vi "Init GUI.vi"(8 "error in (no error)":errorcluster, 11 "Guardian in":refnum<class "Guardian.lvclass">) -> (0 "error out":errorcluster, 3 "Guardian out":refnum<class "Guardian.lvclass">)   [LabVIEW 2026, in "TALOS.lvlib" / "Guardian.lvlib" / "Guardian.lvclass"]
uses:
  Guardian.lvclass
  C:/LabVIEW Code/TALOS/talos/Ancestor/Ancestor/Ancestor.lvclass
  C:/LabVIEW Code/TALOS/builds/Actor Framework PPL/Actor Framework.lvlibp/1abvi3w/vi.lib/ActorFramework/Actor/Actor.lvclass
  Ancestor/Ancestor/Ancestor.lvclass/Ancestor.ctl
  Guardian.lvclass/Guardian.ctl
  Guardian Messages/Launch uService Msg/Launch uService Msg.lvclass/Launch uService Msg.ctl
  Guardian Messages/Message to uService Msg/Message to uService Msg.lvclass/Message to uService Msg.ctl
  Ancestor/Ancestor/Read ID.vi
  Support VIs/Generate Error.vi
  FGV/Error Memory/Get Error Description.vi
  Support VIs/Get PC name.vi
  Support VIs/Get Class Name.vi
  <vilib>/Utility/error.llb/Clear Errors.vi
  FGV/Error Memory/Error Memory Core.vi
  <vilib>/AdvancedString/Delimited String to 1D String Array.vi
  <vilib>/AdvancedString/Delimited String to 1D String Array (string).vi
  Support VIs/Circus Root Path.vi
  FGV/Error Memory/Error Crt Lvl checker.vi
  FGV/Error Memory/Error Memory Core.vi/40c8088d-b597-4017-91af-faa98e00292e.vi
  FGV/Error Memory/Error Memory Core.vi/d4a3ab98-063c-4e44-b43d-fbdcfe6c2be2.vi
  Support VIs/Global Constants.vi
  builds/Actor Framework PPL/Actor Framework.lvlibp/1abvi3w/vi.lib/ActorFramework/Message Enqueuer/Enqueue.vi
  Support VIs/Global Memory.vi
  <vilib>/Utility/LVClass/Get LV Class Name.vi
  Support VIs/Is in Packed Library.vi
  Support VIs/TALOS Root path.vi
  Support VIs/Read CSV worksheet.vi
  <vilib>/Utility/error.llb/General Error Handler.vi
  Support VIs/Error Log.vi
  Guardian Messages/Launch uService Msg/Launch uService Msg.lvclass
  Guardian Messages/Message to uService Msg/Message to uService Msg.lvclass
  Ancestor/Ancestor/Ancestor.lvclass
  <vilib>/Comparison/Equal/Equal Functor/Equal Functor.lvclass
  builds/Actor Framework PPL/Actor Framework.lvlibp/1abvi3w/vi.lib/ActorFramework/Actor/Actor.lvclass
  TALOS.lvlib
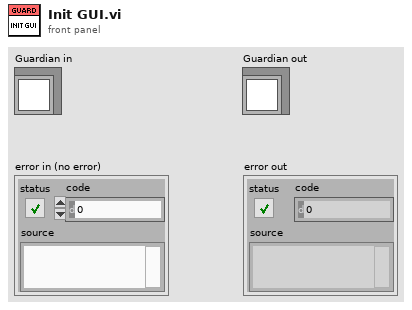
[diagram p1: front panel]
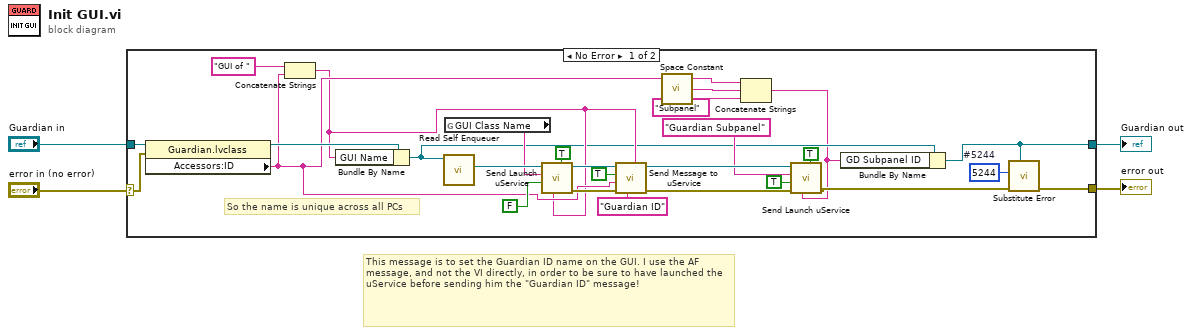
[diagram p0: block diagram]
diagram:
  # "This message is to set the Guardian ID name on the GUI. I use the AF message, and not the VI directly, in order to be sure to have launched the uService before sending him the \"Guardian ID\" message!"
  n1 = case shown="No Error" "error in (no error)" {
    selector: "error in (no error)" -> [w25 w32]
    tunnel: "Guardian in" -> [w27 w33]
    tunnel: [w6 w33] -> w2
    tunnel: [w8 w32] -> w1
    frame No Error {
      w10 = 5244  # #5244
      # "So the name is unique across all PCs"
      n2 = property class="Guardian.lvclass"(reference=w27, error in=w25) -> (reference out=w26:refnum<class "Guardian.lvclass">, "Accessors:ID"=w17:string)  [unwired: 1 out]
      n3 = Concatenate Strings("GUI of ", w17) -> (w13:string)
      n4 = Bundle By Name(cluster=w26, "GUI Name"=w13) -> (w7:refnum<class "Guardian.lvclass">)
      n5 = call "Read Self Enqueuer.vi"("Actor"=w7) -> ("Self Enqueuer"=w30:refnum<class "Message Enqueuer.lvclass">)  [unwired: 10 in]
      n6 = global read "Global Constants.vi" "GUI Class Name"() -> (w29:string)
      n7 = call "Send Launch uService.vi"("Highlander?"=TRUE, "uService ID"=w13, "GUI?"=FALSE, "uService Class Name"=w29, "Message Enqueuer"=w30) -> ("error out"=w23:errorcluster, "Message Enqueuer out"=w24:refnum<class "Message Enqueuer.lvclass">)  [unwired: 5 in]
      n8 = call "Send Message to uService.vi"("uService ID"=w13, "Message"="Guardian ID", "error in (no error)"=w23, "Data"=w17, "Locale?"=TRUE, "Message Enqueuer"=w24) -> ("error out"=w20:errorcluster, "Message Enqueuer out"=w19:refnum<class "Message Enqueuer.lvclass">)  [unwired: 4 in]
      n9 = call <vilib>:"Space Constant.vi"() -> ("String"=w14:string)
      n10 = Concatenate Strings(w17, w14, "Subpanel" ("string")) -> (w5:string)
      n11 = call "Send Launch uService.vi"("Highlander?"=TRUE, "uService ID"=w5, "error in (no error)"=w20, "GUI?"=TRUE, "uService Class Name"="Guardian Subpanel", "Message Enqueuer"=w19) -> ("error out"=w9:errorcluster)  [unwired: 4 in, 1 out]
      n12 = Bundle By Name(cluster=w7, "GD Subpanel ID"=w5) -> (w6:refnum<class "Guardian.lvclass">)
      n13 = call "Substitute Error.vi"("LabVIEW Object"=w6, "error in (no error)"=w9, "Error Code"=w10) -> ("error out"=w8:errorcluster)  [unwired: 8 in]
    }
    frame Error {
    }
  }
  "Guardian out" <- w2
  "error out" <- w1
